vi "Update Fix Button.vi"(7 "Fix It Button Ref":refnum<vi>, 8 "Error In":errorcluster, 10 "Warning Index":i32, 11 "Warnings":T1[](array[typedef])) -> (0 "Error Out":errorcluster, 3 "Warnings":T1[](array[typedef]))   [LabVIEW 2014, in "LMH-LINX.lvlib"]
uses:
  <vilib>/MakerHub/LINX/LMH-LINX.lvlib
  <vilib>/MakerHub/LINX/Private/Utilties/Target Management/Target Compatibility Warnings.ctl
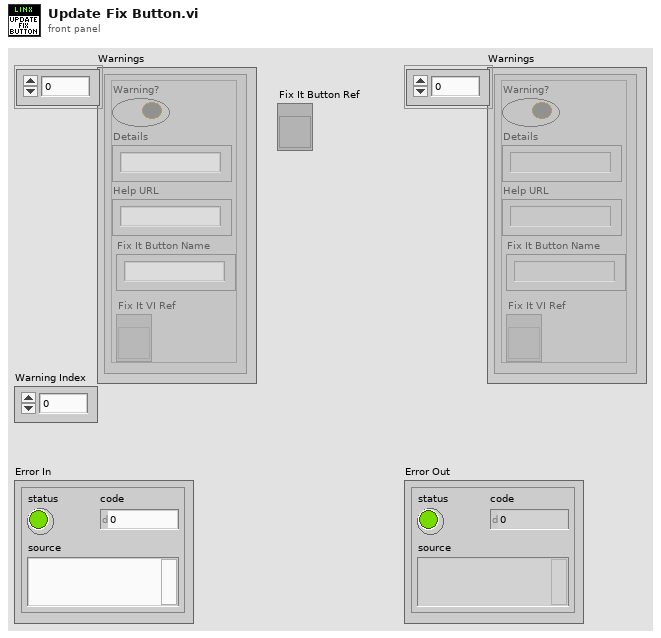
[diagram p1: front panel]
types:
  T1 = typedef "LMH-LINX.lvlib/Target Compatibility Warnings.ctl" = cluster{"Warning?":bool, "Details":string, "Help URL":string, "Fix It Button Name":string, "Fix It VI Ref":refnum<vi>}
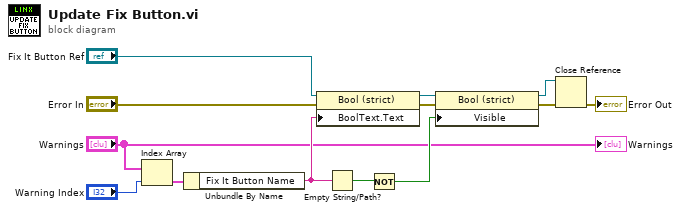
[diagram p0: block diagram]
diagram:
  n1 = Index Array(array="Warnings", index="Warning Index") -> (element=w12:T1)
  n2 = Unbundle By Name(w12) -> ("Fix It Button Name"=w9:string)
  n3 = property on="Property Node" class="Bool (strict)"(reference="Fix It Button Ref", error in="Error In", "BoolText.Text"=w9) -> (reference out=w3:refnum<vi>, error out=w8:errorcluster)
  n4 = Empty String/Path?(string/path=w9) -> (empty?=w7:bool)
  n5 = Not(x=w7) -> (.not. x?=w6:bool)
  n6 = property on="Property Node" class="Bool (strict)"(reference=w3, error in=w8, "Visible"=w6) -> (reference out=w4:refnum<vi>, error out=w5:errorcluster)
  n7 = Close Reference(reference=w4, error in (no error)=w5) -> (error out=→"Error Out":errorcluster)
  "Warnings" <- "Warnings"
